vi "Import From Config.vi"(7 "selected path":path, 8 "error in":errorcluster, 9 "Overwrite Existing Channels?":bool=TRUE, 10 "Overwrite Device Settings?":bool=TRUE, 11 "Device Ref in":T1 format="%.0x") -> (0 "error out":errorcluster)   [LabVIEW 2015, in "Modbus Master System Explorer.lvlib"]
uses:
  Modbus Master System Explorer.lvlib
  <vilib>/NI Veristand/Custom Device API/Custom Device Item Ref.ctl
  Modbus Type.ctl
  Shared/Controls/Data Model/Mapping.ctl
  Shared/Controls/Data Model/DataType.ctl
  <vilib>/NI Veristand/Custom Device API/Custom Device Channel Type.ctl
  Shared/Constants.vi
  <vilib>/NI Veristand/Custom Device Tools/Custom Device Utility Library/NI VeriStand - Search for Item by GUID.vi
  <vilib>/Utility/config.llb/Read Key (String).vi
  <vilib>/Utility/config.llb/Read Key (U32).vi
  <vilib>/NI Veristand/Custom Device Tools/Custom Device Utility Library/NI VeriStand - Search for Item by Name.vi
  <vilib>/Utility/config.llb/NI_LVConfig.lvlib
  Shared/Modbus Master Shared.lvlib
  <vilib>/NI VeriStand/Custom Device Tools/Custom Device Utility Library/Custom Device Utility Library.lvlib
  <vilib>/NI VeriStand/Custom Device API/Custom Device API.lvlib
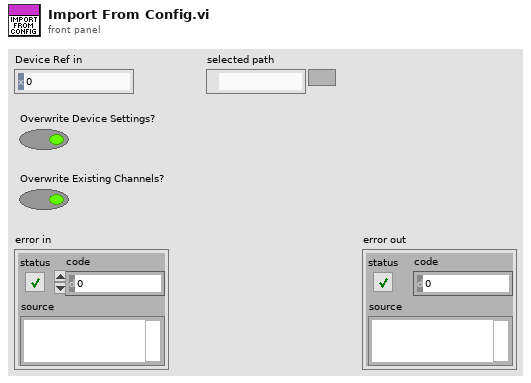
[diagram p1: front panel]
types:
  T1 = typedef "Custom Device API.lvlib/Custom Device Item Ref.ctl" = u64
  T2 = typedef "Custom Device API.lvlib/Custom Device Channel Type.ctl" = enum16{"Input", "Output"}
  T3 = typedef "Modbus Master Shared.lvlib/Mapping.ctl" = cluster{"DataType":T4, "Starting Address":u16, "Sub-Index (Bool)":u16, "VS Reference":T1}
  T4 = typedef "Modbus Master Shared.lvlib/DataType.ctl" = enum16{"Double", "Single", "I64", "I32", "I16", "I8", "U64", "U32", "U16", "U8", "Boolean"}
  T5 = typedef "NI_LVConfig.lvlib/Config Data RefNum.ctl" = refnum<k1>
  T6 = typedef "Modbus Master Shared.lvlib/Modbus Type.ctl" = enum16{"Coil", "Discrete Input", "Holding Register", "Input Register"}
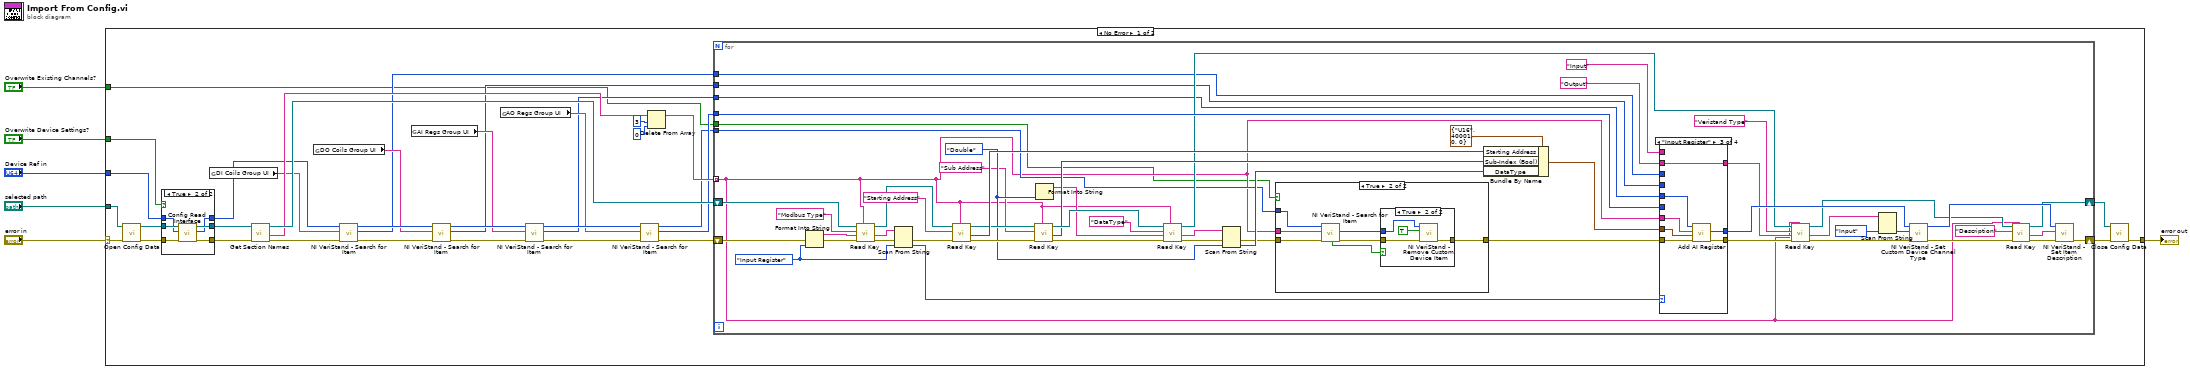
[diagram p0: block diagram]
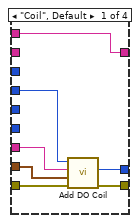
[diagram p5: hidden frame]
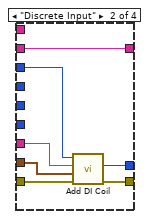
[diagram p6: hidden frame]
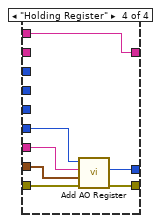
[diagram p7: hidden frame]
diagram:
  n1 = case shown="No Error" "error in" {
    selector: "error in" -> [w31 w147]
    tunnel: "selected path" -> [w41 _]
    tunnel: [w40 w147] -> w5
    tunnel: "Device Ref in" -> [w38 _]
    tunnel: "Overwrite Device Settings?" -> [w9 _]
    tunnel: "Overwrite Existing Channels?" -> [w7 _]
    frame No Error {
      n2 = call <vilib>:"Open Config Data.vi"("error in (no error)"=w31, "configuration file path"=w41) -> ("error out"=w30:errorcluster, "refnum"=w39:T5)  [unwired: 7 in, 1 out]
      n3 = case shown="True" w9 {
        tunnel: w39 -> [w42 w50]
        tunnel: w38 -> [w44 w49]
        tunnel: [w42 w48] -> w37
        tunnel: w30 -> [w43 w47]
        tunnel: [w43 w46] -> w29
        tunnel: [w44 w45] -> w15
        frame False {
        }
        frame True {
          n4 = call "Config Read Interface.vi"("error in (no error)"=w47, "Device Ref in"=w49, "Refnum in"=w50) -> ("error out"=w46:errorcluster, "Device Ref out"=w45:T1, "Refnum out"=w48:T5)  [unwired: 6 in]
        }
      }
      n5 = global read "Constants.vi" "DI Coils Group UI"() -> (w14:string)
      n6 = call <vilib>:"Get Section Names.vi"("error in (no error)"=w29, "refnum"=w37) -> ("error out"=w17:errorcluster, "section names"=w32:string[], "refnum out"=w34:T5)  [unwired: 7 in]
      n7 = global read "Constants.vi" "DO Coils Group UI"() -> (w20:string)
      n8 = call-poly <vilib>:"NI VeriStand - Search for Item.vi"("error in"=w17, "Item GUID"=w14, "Section Ref in"=w15) -> ("error out"=w22:errorcluster, "Item Ref"=w12:T1, "Section Ref out"=w21:T1)  [unwired: 5 in, 1 out]
      n9 = global read "Constants.vi" "AI Regs Group UI"() -> (w19:string)
      n10 = call-poly <vilib>:"NI VeriStand - Search for Item.vi"("error in"=w22, "Item GUID"=w20, "Section Ref in"=w21) -> ("error out"=w25:errorcluster, "Item Ref"=w13:T1, "Section Ref out"=w23:T1)  [unwired: 5 in, 1 out]
      n11 = global read "Constants.vi" "AO Regs Group UI"() -> (w18:string)
      n12 = call-poly <vilib>:"NI VeriStand - Search for Item.vi"("error in"=w25, "Item GUID"=w19, "Section Ref in"=w23) -> ("error out"=w26:errorcluster, "Item Ref"=w10:T1, "Section Ref out"=w24:T1)  [unwired: 5 in, 1 out]
      n13 = call-poly <vilib>:"NI VeriStand - Search for Item.vi"("error in"=w26, "Item GUID"=w18, "Section Ref in"=w24) -> ("error out"=w16:errorcluster, "Item Ref"=w11:T1, "Section Ref out"=w8:T1)  [unwired: 5 in, 1 out]
      n14 = Delete From Array(array=w32, length=3, index=0) -> (array with subset deleted=w33:string[])  [unwired: 1 out]
      n15 = for {
        tunnel: w33 -> [w54] mode=indexing
        shift-right: [w62] -> w27
        shift-left: w16 -> [w69]
        shift-right: [w58] -> w28
        shift-left: w34 -> [w70]
        tunnel: w13 -> [w80]
        tunnel: w12 -> [w81]
        tunnel: w11 -> [w103]
        tunnel: w10 -> [w79]
        tunnel: w8 -> [w55]
        tunnel: w7 -> [w53]
        w72 = DataType."Double" ("DataType")
        w74 = Modbus_Type."Input Register" ("Type")
        n16 = Format Into String(error in=w69, w74) -> (resulting string=w73:string, error out=w68:errorcluster)  [unwired: 2 in]
        n17 = call-poly <vilib>:"Read Key.vi"("section"=w54, "error in (no error)"=w68, "default value"=w73, "key"="Modbus Type", "refnum"=w70) -> ("error out"=w105:errorcluster, "value"=w104:string, "refnum out"=w102:T5)  [unwired: 3 in, 1 out]
        n18 = Scan From String(input string=w104, error in=w105, default 1=w74) -> (error out=w101:errorcluster, output 1=w82:T6)  [unwired: 2 in, 2 out]
        n19 = call-poly <vilib>:"Read Key.vi"("section"=w54, "error in (no error)"=w101, "key"="Starting Address", "refnum"=w102) -> ("error out"=w94:errorcluster, "value"=w99:u32, "refnum out"=w97:T5)  [unwired: 4 in, 1 out]
        n20 = call-poly <vilib>:"Read Key.vi"("section"=w54, "error in (no error)"=w94, "key"="Sub Address", "refnum"=w97) -> ("error out"=w96:errorcluster, "value"=w93:u32, "refnum out"=w95:T5)  [unwired: 4 in, 1 out]
        n21 = Format Into String(w72) -> (resulting string=w71:string)  [unwired: 3 in, 1 out]
        n22 = call-poly <vilib>:"Read Key.vi"("section"=w54, "error in (no error)"=w96, "default value"=w71, "key"="DataType", "refnum"=w95) -> ("error out"=w91:errorcluster, "value"=w92:string, "refnum out"=w86:T5)  [unwired: 3 in, 1 out]
        n23 = Scan From String(input string=w92, error in=w91, default 1=w72) -> (error out=w52:errorcluster, output 1=w90:T4)  [unwired: 2 in, 2 out]
        n24 = case shown="True" w53 {
          tunnel: w55 -> [_ w113]
          tunnel: w54 -> [_ w112]
          tunnel: w52 -> [w106 w108]
          tunnel: [w106 w107] -> w51
          frame False {
          }
          frame True {
            n25 = call-poly <vilib>:"NI VeriStand - Search for Item.vi"("error in"=w108, "Item Name"=w112, "Section Ref in"=w113) -> ("error out"=w109:errorcluster, "Item Ref"=w110:T1, "Found"=w111:bool)  [unwired: 5 in, 1 out]
            n26 = case shown="True" w111 {
              tunnel: w110 -> [_ w118]
              tunnel: w109 -> [w114 w117]
              tunnel: [w114 w116] -> w107
              frame False {
              }
              frame True {
                n27 = call <vilib>:"NI VeriStand - Remove Custom Device Item.vi"("error in (no error)"=w117, "Force Delete (F)"=TRUE, "Item Ref in"=w118) -> ("error out"=w116:errorcluster)  [unwired: 7 in, 1 out]
              }
            }
          }
        }
        n28 = Bundle By Name(cluster=T3 {"DataType"=enum."U16", "Starting Address"=40001, "Sub-Index (Bool)"=0, "VS Reference"=0} ("Mapping"), "Starting Address"=w99, "Sub-Index (Bool)"=w93, "DataType"=w90) -> (w98:T3)
        n29 = case shown="\"Input Register\"" w82 {
          tunnel: w103 -> [_ _ _ w146]
          tunnel: w54 -> [w122 w128 w134 w145]
          tunnel: w98 -> [w123 w129 w139 w144]
          tunnel: w51 -> [w125 w132 w133 w143]
          tunnel: [w121 w130 w137 w142] -> w89
          tunnel: [w124 w131 w138 w141] -> w88
          tunnel: w81 -> [_ w127 _ _]
          tunnel: w80 -> [w120 _ _ _]
          tunnel: w79 -> [_ _ w135 _]
          tunnel: [w119 w126 w136 w140] -> w77
          tunnel: "Input" ("default value") -> [w119 _ _ w140]
          tunnel: "Output" ("default value") -> [_ w126 w136 _]
          frame "Coil", Default {
            n30 = call "Add DO Coil.vi"("error in (no error)"=w125, "Mapping"=w123, "Label"=w122, "Node Ref In"=w120) -> ("error out"=w124:errorcluster, "Channel Ref"=w121:T1)  [unwired: 5 in, 1 out]
          }
          frame "Discrete Input" {
            n31 = call "Add DI Coil.vi"("error in (no error)"=w132, "Mapping"=w129, "Label"=w128, "Node Ref In"=w127) -> ("error out"=w131:errorcluster, "Channel Ref Out"=w130:T1)  [unwired: 5 in, 1 out]
          }
          frame "Input Register" {
            n32 = call "Add AI Register.vi"("error in (no error)"=w133, "Mapping"=w139, "Label"=w134, "Node Ref In"=w135) -> ("error out"=w138:errorcluster, "Channel Ref out"=w137:T1)  [unwired: 5 in, 1 out]
          }
          frame "Holding Register" {
            n33 = call "Add AO Register.vi"("error in (no error)"=w143, "Mapping"=w144, "Label"=w145, "Node Ref In"=w146) -> ("error out"=w141:errorcluster, "Channel Ref out"=w142:T1)  [unwired: 5 in, 1 out]
          }
        }
        n34 = call-poly <vilib>:"Read Key.vi"("section"=w54, "error in (no error)"=w88, "default value"=w77, "key"="Veristand Type", "refnum"=w86) -> ("error out"=w87:errorcluster, "value"=w84:string, "refnum out"=w59:T5)  [unwired: 3 in, 1 out]
        n35 = Scan From String(input string=w84, default 1=Custom_Device_Channel_Type."Input" ("Type")) -> (output 1=w83:T2)  [unwired: 3 in, 3 out]
        n36 = call <vilib>:"NI VeriStand - Set Custom Device Channel Type.vi"("error in (no error)"=w87, "Type"=w83, "Channel Ref in"=w89) -> ("error out"=w61:errorcluster, "Channel Ref out"=w63:T1)  [unwired: 7 in]
        n37 = call-poly <vilib>:"Read Key.vi"("section"=w54, "error in (no error)"=w61, "key"="Description", "refnum"=w59) -> ("error out"=w60:errorcluster, "value"=w56:string, "refnum out"=w58:T5)  [unwired: 4 in, 1 out]
        n38 = call <vilib>:"NI VeriStand - Set Item Description.vi"("error in (no error)"=w60, "Description"=w56, "Item Ref in"=w63) -> ("error out"=w62:errorcluster)  [unwired: 6 in, 2 out]
      }
      n39 = call <vilib>:"Close Config Data.vi"("error in (no error)"=w27, "refnum"=w28) -> ("error out"=w40:errorcluster)  [unwired: 8 in, 1 out]
    }
    frame Error {
    }
  }
  "error out" <- w5
